vi "Chop One Bin (VI).vi"(4 "tolerance":dbl=1e-16, 6 "data":variant, 7 "f(x)":refnum<vi>, 8 "error in (no error)":errorcluster, 10 "chop?":bool, 11 "bin":cluster{"lower limit":dbl, "upper limit":dbl}) -> (0 "error out":errorcluster, 2 "Chop Out":bool[](array[boolean]), 3 "Bins Out":cluster{"lower limit":dbl, "upper limit":dbl}[](array[cluster]))   [LabVIEW 2019]
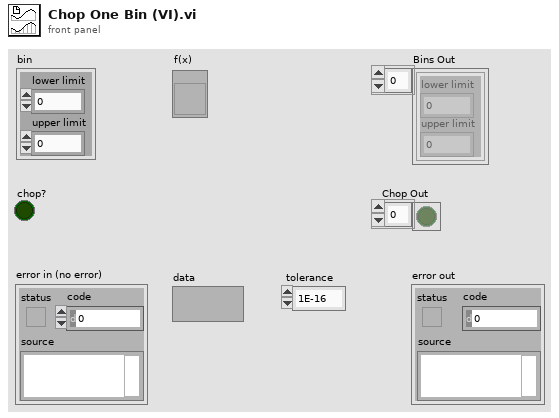
[diagram p1: front panel]
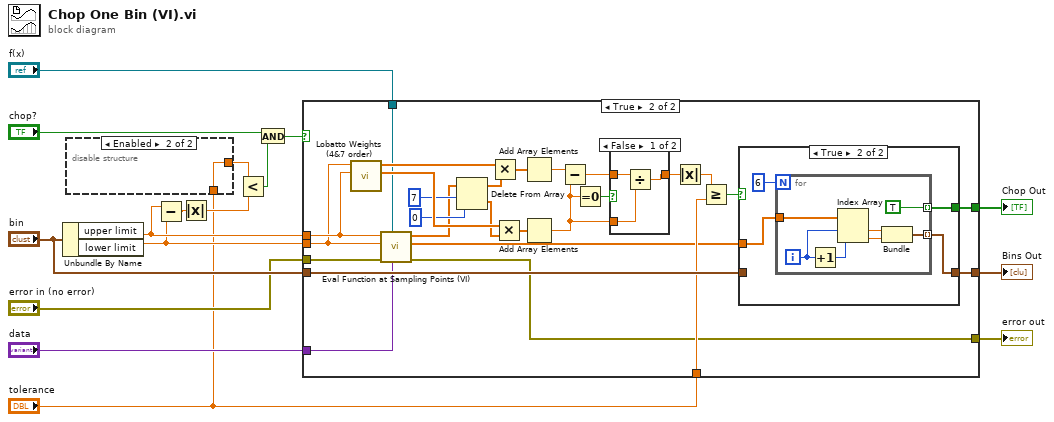
[diagram p0: block diagram]
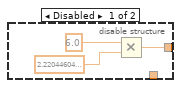
[diagram p2: hidden frame]
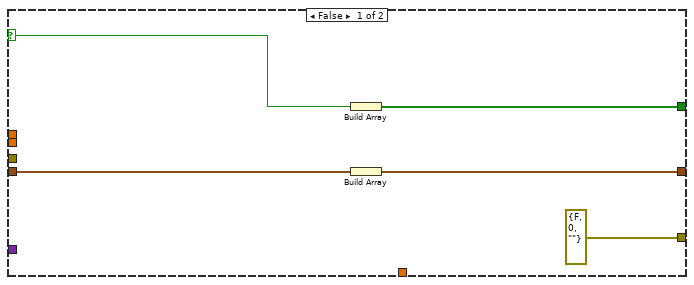
[diagram p3: hidden frame]
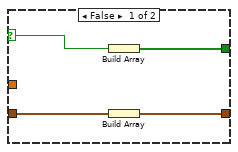
[diagram p5: hidden frame]
diagram:
  n1 = Unbundle By Name("bin") -> ("upper limit"=w11:dbl, "lower limit"=w10:dbl)
  n2 = disable-structure shown="Enabled" {
    disable-tunnel: [w17 w20] -> w7
    disable-tunnel: "tolerance" -> [_ w20]
    frame Disabled {
      n3 = Multiply(x=6.0, y=2.220446049250313e-16 ("x^y")) -> (x*y=w17:dbl)
    }
    frame Enabled {
    }
  }
  n4 = Subtract(x=w11, y=w10) -> (x-y=w13:dbl)
  n5 = Absolute Value(x=w13) -> (abs(x)=w8:dbl)
  n6 = Less?(x=w7, y=w8) -> (x < y?=w6:bool)
  n7 = And(x="chop?", y=w6) -> (x .and. y?=w9:bool)
  n8 = case shown="True" w9 {
    selector: w9 -> [w25 _]
    tunnel: [w22 w46] -> w16
    tunnel: [w24 w45] -> w15
    tunnel: "bin" -> [w23 w44]
    tunnel: w11 -> [_ w33]
    tunnel: w10 -> [_ w32]
    tunnel: "tolerance" -> [_ w43]
    tunnel: [errorcluster {"status"=FALSE, "code"=0, "source"=""} ("error out") w31] -> w5
    tunnel: "f(x)" -> [_ w28]
    tunnel: "data" -> [_ w27]
    tunnel: "error in (no error)" -> [_ w26]
    frame False {
      n9 = Build Array(w25) -> (w24:bool[])
      n10 = Build Array(w23) -> (w22:cluster{"lower limit":dbl, "upper limit":dbl}[])
    }
    frame True {
      n11 = call "Lobatto Weights (4&7 order).vi"("lower limit"=w33, "upper limit"=w32) -> ("Weights (7-Order)"=w51:dbl[], "Weights (4-Order)"=w52:dbl[])  [unwired: 8 in]
      n12 = call "Eval Function at Sampling Points (VI).vi"("data"=w27, "f(x)"=w28, "error in (no error)"=w26, "lower limit"=w32, "upper limit"=w33) -> ("error out"=w31:errorcluster, "Sampling points (7-order)"=w30:dbl[], "Function Evaluations (7 and 4 pts)"=w29:dbl[])  [unwired: 4 in]
      n13 = Delete From Array(array=w29, length=7, index=0) -> (deleted portion=w34:dbl[], array with subset deleted=w35:dbl[])
      n14 = Multiply(x=w52, y=w35) -> (x*y=w50:dbl[])
      n15 = Multiply(x=w51, y=w34) -> (x*y=w49:dbl[])
      n16 = Add Array Elements(numeric array=w50) -> (sum=w48:dbl)
      n17 = Add Array Elements(numeric array=w49) -> (sum=w40:dbl)
      n18 = Subtract(x=w48, y=w40) -> (x-y=w41:dbl)
      n19 = Equal To 0?(x=w40) -> (x = 0?=w42:bool)
      n20 = case shown="False" w42 {
        tunnel: w41 -> [w55 w56]
        tunnel: w40 -> [w54 _]
        tunnel: [w53 w56] -> w39
        frame False {
          n21 = Divide(x=w55, y=w54) -> (x/y=w53:dbl)
        }
        frame True {
        }
      }
      n22 = Absolute Value(x=w39) -> (abs(x)=w38:dbl)
      n23 = Greater Or Equal?(x=w38, y=w43) -> (x >= y?=w47:bool)
      n24 = case shown="True" w47 {
        selector: w47 -> [w58 _]
        tunnel: w30 -> [_ w63]
        tunnel: [w59 w62] -> w46
        tunnel: w44 -> [w60 _]
        tunnel: [w57 w61] -> w45
        frame False {
          n25 = Build Array(w58) -> (w57:bool[])
          n26 = Build Array(w60) -> (w59:cluster{"lower limit":dbl, "upper limit":dbl}[])
        }
        frame True {
          n27 = for {
            N: 6 -> [_]
            tunnel: w63 -> [w71]
            tunnel: [w66] -> w62 mode=indexing
            tunnel: [TRUE] -> w61 mode=indexing
            i -> [w70]
            n28 = Increment(x=w70) -> (x+1=w69:i32)
            n29 = Index Array(array=w71, index #1=w70, index #2=w69) -> (element #1=w67:dbl, element #2=w68:dbl)
            n30 = Bundle(w67, w68) -> (w66:cluster{dbl, dbl})  [unwired: 1 in]
          }
        }
      }
    }
  }
  "Bins Out" <- w16
  "Chop Out" <- w15
  "error out" <- w5
